vi "FPGA_ScanningPreview.vi"() -> ()   [LabVIEW 2024]
uses:
  <vilib>/rvi/Emulation/niFpgaSctlEmulationGetInTimedLoop.vi
  <vilib>/rvi/Emulation/niFpgaProcessEmulError.vi
  <vilib>/rvi/eio/common/nirviEmuTemplateMethod_errors.vi
  <vilib>/rvi/Emulation/niFpgaEmulationIsFPGAContextNoSignature.vi
  <vilib>/rvi/DataTransferAndStorage/Container/Common/niFpgaContainerGetUniqueNameForEmu.vi
  <vilib>/rvi/Memory/Memory_Emulation/niFpgaMemoryEmulationCacheClearOnFirstRun.vi
  <vilib>/rvi/Memory/Memory_Emulation/nirvimemoryEmulationManagerCache_MakeExclusive.vi
  <vilib>/rvi/Memory/Memory_Emulation/niFpgaMemoryEmulationValidateCache.vi
  <vilib>/rvi/Memory/Memory_Emulation/nirvimemoryEmulationManagerCache_InsertValue.vi
  <vilib>/Utility/error.llb/Clear Errors.vi
  <vilib>/rvi/Memory/Memory_Emulation/nirvimemoryEmulationManagerCache_ReleaseExclusive.vi
  <vilib>/rvi/Memory/Memory_Emulation/nirvimemoryEmulationManagerCache_GetValue.vi
  <vilib>/rvi/Memory/Memory_Emulation/nirvimemoryEmulationManagerCache_SetValue.vi
  <vilib>/rvi/Emulation/niFpgaGetClockAttributes.vi
  <vilib>/rvi/Emulation/niFpgaEmulationReportErrorSimple.vi
  <vilib>/rvi/Emulation/niFpgaCriticalErrorInLSC.vi
  <vilib>/eio/EIONode/EIONode.xnode
  <vilib>/rvi/DataTransferAndStorage/Container/XNode/niFpgaContainer.xnode
  <vilib>/rvi/DataTransferAndStorage/Register/Emulation/niFpgaRegisterEmulation.vi
  <vilib>/rvi/FXPMathLib/FxpAdd/XNode/nifxpmath_Add.xnode
  <vilib>/rvi/FXPMathLib/FxpSub/XNode/nifxpmath_Sub.xnode
  <vilib>/rvi/FXPMathLib/sim/FxpSim.dll
panel:
  in  "rate us":i32
  out "TargetDone?":bool
  out "ScanFinished?":bool
  in  "stop":bool
  in  "Y_end":fxp<+/-,48,16>
  in  "Y_start":fxp<+/-,48,16>
  in  "X_end":fxp<+/-,48,16>
  in  "X_start":fxp<+/-,48,16>
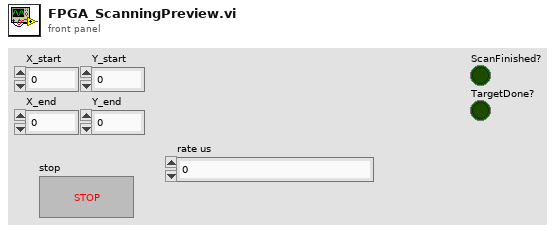
[diagram p1: front panel]
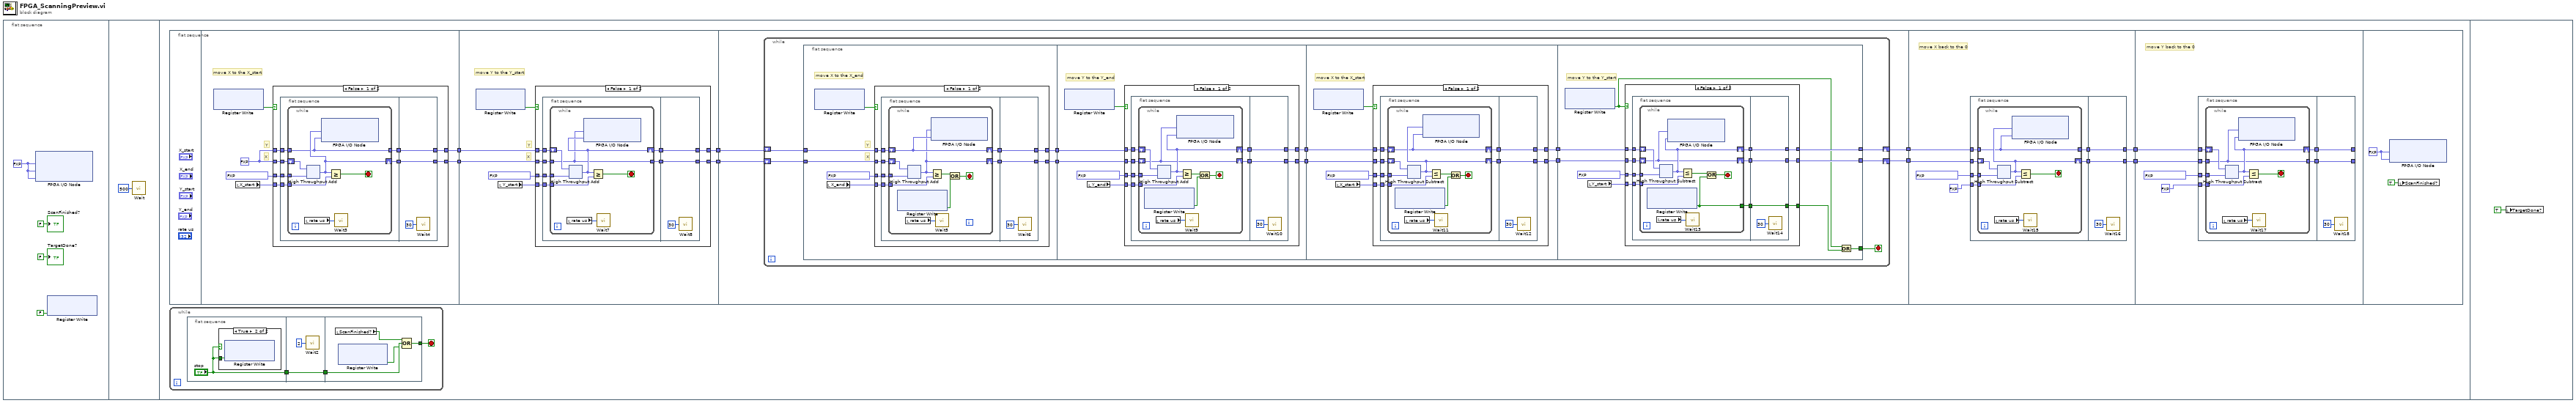
[diagram p0: block diagram]
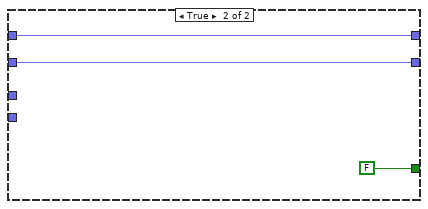
[diagram p8: hidden frame]
diagram:
  n1 = flat-sequence {
    frame #0 {
      w4 = fxp<+/-,20,5> 0.0 ("Connector0/AO0")
      n2 = xnode "FPGA I/O Node"("Connector0/AO0"=w4, "Connector0/AO1"=w4, "Connector0/AO2"=w4) -> ()  [unwired: 3 in, 3 out]
      n3 = xnode ("Register Write")("Data"=FALSE) -> ()  [unwired: 1 in, 1 out]
      "ScanFinished?" <- FALSE
      "TargetDone?" <- FALSE
    }
    frame #1 {
      n4 = call "Wait"("Count(mSec)"=u16 500) -> ()  [unwired: 1 out]
    }
    frame #2 {
      n5 = flat-sequence {
        tunnel: [w27] -> w13
        tunnel: [w25] -> w11
        tunnel: w13 -> [w59]
        tunnel: [w57] -> w12
        tunnel: w11 -> [w60]
        tunnel: [w58] -> w10
        tunnel: w10 -> [w93]
        tunnel: w12 -> [w92]
        tunnel: [w91] -> w9
        tunnel: [w90] -> w8
        tunnel: w9 -> [w258]
        tunnel: w8 -> [w257]
        tunnel: [w254] -> w7
        tunnel: [w253] -> w6
        tunnel: w7 -> [w278]
        tunnel: w6 -> [w277]
        frame #0 {
        }
        frame #1 {
          w26 = fxp<+/-,48,16> 0.0 ("y")
          # "X"
          # "Y"
          # "move X to the X_start"
          n6 = xnode ("Register Write")() -> ("Data"=w30:bool)  [unwired: 1 in, 1 out]
          n7 = local read "X_start"() -> (w28:fxp<+/-,48,16>)
          n8 = case shown="False" w30 {
            tunnel: w26 -> [w38 w56]
            tunnel: fxp<+/-,48,16> 0.00030517578125 ("y") -> [w37 _]
            tunnel: w28 -> [w36 _]
            tunnel: [w34 w56] -> w27
            tunnel: w26 -> [w33 w55]
            tunnel: [w31 w55] -> w25
            frame False {
              n9 = flat-sequence {
                tunnel: w38 -> [w42]
                tunnel: w37 -> [w44]
                tunnel: w36 -> [w43]
                tunnel: [w41] -> w35
                tunnel: w33 -> [w40]
                tunnel: [w39] -> w32
                tunnel: w35 -> [w53]
                tunnel: [w53] -> w34
                tunnel: w32 -> [w52]
                tunnel: [w52] -> w31
                frame #0 {
                  n10 = while {
                    tunnel: w44 -> [w51]
                    tunnel: w43 -> [w50]
                    shift-right: [w47] -> w41
                    shift-left: w42 -> [w48]
                    tunnel: w40 -> [w45]
                    tunnel: [w45] -> w39
                    stop <- w46 stop-if-true
                    n11 = local read "rate us"() -> (w49:i32)
                    n12 = xnode ("High Throughput Add")("x"=w48, "y"=w51) -> ("x+y"=w47:fxp<+/-,48,16>)
                    n13 = xnode "FPGA I/O Node"("Connector0/AO0"=w47, "Connector0/AO1"=w45) -> ()  [unwired: 2 in, 2 out]
                    n14 = Greater Or Equal?(x=w47, y=w50) -> (x >= y?=w46:bool)
                    n15 = call "Wait3"("Count(uSec)"=w49) -> ()  [unwired: 1 out]
                  }
                }
                frame #1 {
                  n16 = call "Wait4"("Count(uSec)"=u8 30) -> ()  [unwired: 1 out]
                }
              }
            }
            frame True {
            }
          }
        }
        frame #2 {
          # "X"
          # "Y"
          # "move Y to the Y_start"
          n17 = xnode ("Register Write")() -> ("Data"=w61:bool)  [unwired: 1 in, 1 out]
          n18 = local read "Y_start"() -> (w63:fxp<+/-,48,16>)
          n19 = case shown="False" w61 {
            tunnel: w59 -> [w71 w89]
            tunnel: fxp<+/-,48,16> 0.00030517578125 ("y") -> [w70 _]
            tunnel: w63 -> [w69 _]
            tunnel: [w67 w89] -> w57
            tunnel: w60 -> [w66 w88]
            tunnel: [w64 w88] -> w58
            frame False {
              n20 = flat-sequence {
                tunnel: w71 -> [w75]
                tunnel: w70 -> [w77]
                tunnel: w69 -> [w76]
                tunnel: [w74] -> w68
                tunnel: w66 -> [w73]
                tunnel: [w72] -> w65
                tunnel: w68 -> [w86]
                tunnel: [w86] -> w67
                tunnel: w65 -> [w85]
                tunnel: [w85] -> w64
                frame #0 {
                  n21 = while {
                    tunnel: w77 -> [w84]
                    tunnel: w76 -> [w83]
                    tunnel: w75 -> [w78]
                    tunnel: [w78] -> w74
                    shift-right: [w79] -> w72
                    shift-left: w73 -> [w81]
                    stop <- w80 stop-if-true
                    n22 = local read "rate us"() -> (w82:i32)
                    n23 = xnode ("High Throughput Add")("x"=w81, "y"=w84) -> ("x+y"=w79:fxp<+/-,48,16>)
                    n24 = xnode "FPGA I/O Node"("Connector0/AO0"=w78, "Connector0/AO1"=w79) -> ()  [unwired: 2 in, 2 out]
                    n25 = Greater Or Equal?(x=w79, y=w83) -> (x >= y?=w80:bool)
                    n26 = call "Wait7"("Count(uSec)"=w82) -> ()  [unwired: 1 out]
                  }
                }
                frame #1 {
                  n27 = call "Wait8"("Count(uSec)"=u8 30) -> ()  [unwired: 1 out]
                }
              }
            }
            frame True {
            }
          }
        }
        frame #3 {
          n28 = while {
            shift-right: [w95] -> w90
            shift-left: w92 -> [w101]
            shift-right: [w96] -> w91
            shift-left: w93 -> [w102]
            stop <- w94 stop-if-true
            n29 = flat-sequence {
              tunnel: w102 -> [w108]
              tunnel: w101 -> [w107]
              tunnel: [w106] -> w104
              tunnel: [w105] -> w103
              tunnel: w104 -> [w143]
              tunnel: w103 -> [w142]
              tunnel: [w141] -> w100
              tunnel: [w140] -> w99
              tunnel: w100 -> [w178]
              tunnel: w99 -> [w177]
              tunnel: [w176] -> w98
              tunnel: [w175] -> w97
              tunnel: w98 -> [w216]
              tunnel: w97 -> [w215]
              tunnel: [w214] -> w96
              tunnel: [w213] -> w95
              tunnel: [w210] -> w94
              frame #0 {
                # "X"
                # "Y"
                # "move X to the X_end"
                n30 = xnode ("Register Write")() -> ("Data"=w109:bool)  [unwired: 1 in, 1 out]
                n31 = local read "X_end"() -> (w111:fxp<+/-,48,16>)
                n32 = case shown="False" w109 {
                  tunnel: w107 -> [w119 w139]
                  tunnel: fxp<+/-,48,16> 0.00030517578125 ("y") -> [w118 _]
                  tunnel: w111 -> [w117 _]
                  tunnel: [w115 w139] -> w105
                  tunnel: w108 -> [w114 w138]
                  tunnel: [w112 w138] -> w106
                  frame False {
                    n33 = flat-sequence {
                      tunnel: w119 -> [w123]
                      tunnel: w118 -> [w125]
                      tunnel: w117 -> [w124]
                      tunnel: [w122] -> w116
                      tunnel: w114 -> [w121]
                      tunnel: [w120] -> w113
                      tunnel: w116 -> [w136]
                      tunnel: [w136] -> w115
                      tunnel: w113 -> [w135]
                      tunnel: [w135] -> w112
                      frame #0 {
                        n34 = while {
                          tunnel: w125 -> [w134]
                          tunnel: w124 -> [w133]
                          shift-right: [w126] -> w122
                          shift-left: w123 -> [w131]
                          shift-right: [w130] -> w120
                          shift-left: w121 -> [w130]
                          stop <- w127 stop-if-true
                          n35 = xnode ("Register Write")() -> ("Data"=w128:bool)  [unwired: 1 in, 1 out]
                          n36 = local read "rate us"() -> (w132:i32)
                          n37 = xnode ("High Throughput Add")("x"=w131, "y"=w134) -> ("x+y"=w126:fxp<+/-,48,16>)
                          n38 = Greater Or Equal?(x=w126, y=w133) -> (x >= y?=w129:bool)
                          n39 = xnode "FPGA I/O Node"("Connector0/AO0"=w126, "Connector0/AO1"=w130) -> ()  [unwired: 2 in, 2 out]
                          n40 = call "Wait5"("Count(uSec)"=w132) -> ()  [unwired: 1 out]
                          n41 = Or(x=w129, y=w128) -> (x .or. y?=w127:bool)
                        }
                      }
                      frame #1 {
                        n42 = call "Wait6"("Count(uSec)"=u8 30) -> ()  [unwired: 1 out]
                      }
                    }
                  }
                  frame True {
                  }
                }
              }
              frame #1 {
                # "move Y to the Y_end"
                n43 = xnode ("Register Write")() -> ("Data"=w146:bool)  [unwired: 1 in, 1 out]
                n44 = local read "Y_end"() -> (w144:fxp<+/-,48,16>)
                n45 = case shown="False" w146 {
                  tunnel: w142 -> [w154 w174]
                  tunnel: fxp<+/-,48,16> 0.00030517578125 ("y") -> [w153 _]
                  tunnel: w144 -> [w152 _]
                  tunnel: [w150 w174] -> w140
                  tunnel: w143 -> [w149 w173]
                  tunnel: [w147 w173] -> w141
                  frame False {
                    n46 = flat-sequence {
                      tunnel: w154 -> [w158]
                      tunnel: w153 -> [w160]
                      tunnel: w152 -> [w159]
                      tunnel: [w157] -> w151
                      tunnel: w149 -> [w156]
                      tunnel: [w155] -> w148
                      tunnel: w151 -> [w171]
                      tunnel: [w171] -> w150
                      tunnel: w148 -> [w170]
                      tunnel: [w170] -> w147
                      frame #0 {
                        n47 = while {
                          tunnel: w160 -> [w169]
                          tunnel: w159 -> [w168]
                          shift-right: [w165] -> w155
                          shift-left: w156 -> [w166]
                          shift-right: [w164] -> w157
                          shift-left: w158 -> [w164]
                          stop <- w161 stop-if-true
                          n48 = xnode ("Register Write")() -> ("Data"=w162:bool)  [unwired: 1 in, 1 out]
                          n49 = local read "rate us"() -> (w167:i32)
                          n50 = xnode ("High Throughput Add")("x"=w166, "y"=w169) -> ("x+y"=w165:fxp<+/-,48,16>)
                          n51 = xnode "FPGA I/O Node"("Connector0/AO0"=w164, "Connector0/AO1"=w165) -> ()  [unwired: 2 in, 2 out]
                          n52 = Greater Or Equal?(x=w165, y=w168) -> (x >= y?=w163:bool)
                          n53 = call "Wait9"("Count(uSec)"=w167) -> ()  [unwired: 1 out]
                          n54 = Or(x=w163, y=w162) -> (x .or. y?=w161:bool)
                        }
                      }
                      frame #1 {
                        n55 = call "Wait10"("Count(uSec)"=u8 30) -> ()  [unwired: 1 out]
                      }
                    }
                  }
                  frame True {
                  }
                }
              }
              frame #2 {
                # "move X to the X_start"
                n56 = xnode ("Register Write")() -> ("Data"=w179:bool)  [unwired: 1 in, 1 out]
                n57 = local read "X_start"() -> (w181:fxp<+/-,48,16>)
                n58 = case shown="False" w179 {
                  tunnel: w177 -> [w189 w209]
                  tunnel: fxp<+/-,48,16> 0.00030517578125 ("y") -> [w188 _]
                  tunnel: w181 -> [w187 _]
                  tunnel: [w185 w209] -> w175
                  tunnel: w178 -> [w184 w208]
                  tunnel: [w182 w208] -> w176
                  frame False {
                    n59 = flat-sequence {
                      tunnel: w189 -> [w193]
                      tunnel: w188 -> [w195]
                      tunnel: w187 -> [w194]
                      tunnel: [w192] -> w186
                      tunnel: w184 -> [w191]
                      tunnel: [w190] -> w183
                      tunnel: w186 -> [w206]
                      tunnel: [w206] -> w185
                      tunnel: w183 -> [w205]
                      tunnel: [w205] -> w182
                      frame #0 {
                        n60 = while {
                          tunnel: w195 -> [w201]
                          tunnel: w194 -> [w204]
                          shift-right: [w200] -> w192
                          shift-left: w193 -> [w202]
                          shift-right: [w199] -> w190
                          shift-left: w191 -> [w199]
                          stop <- w196 stop-if-true
                          n61 = xnode ("Register Write")() -> ("Data"=w197:bool)  [unwired: 1 in, 1 out]
                          n62 = local read "rate us"() -> (w203:i32)
                          n63 = xnode "High Throughput Subtract"("x"=w202, "y"=w201) -> ("x-y"=w200:fxp<+/-,48,16>)
                          n64 = xnode "FPGA I/O Node"("Connector0/AO0"=w200, "Connector0/AO1"=w199) -> ()  [unwired: 2 in, 2 out]
                          n65 = Less Or Equal?(x=w200, y=w204) -> (x <= y?=w198:bool)
                          n66 = call "Wait11"("Count(uSec)"=w203) -> ()  [unwired: 1 out]
                          n67 = Or(x=w198, y=w197) -> (x .or. y?=w196:bool)
                        }
                      }
                      frame #1 {
                        n68 = call "Wait12"("Count(uSec)"=u8 30) -> ()  [unwired: 1 out]
                      }
                    }
                  }
                  frame True {
                  }
                }
              }
              frame #3 {
                # "move Y to the Y_start"
                n69 = xnode ("Register Write")() -> ("Data"=w212:bool)  [unwired: 1 in, 1 out]
                n70 = local read "Y_start"() -> (w217:fxp<+/-,48,16>)
                n71 = case shown="False" w212 {
                  tunnel: w215 -> [w228 w251]
                  tunnel: fxp<+/-,48,16> 0.00030517578125 ("y") -> [w227 _]
                  tunnel: w217 -> [w226 _]
                  tunnel: [w224 w251] -> w213
                  tunnel: w216 -> [w223 w250]
                  tunnel: [w221 w250] -> w214
                  tunnel: [w219 FALSE ("Data")] -> w211
                  frame False {
                    n72 = flat-sequence {
                      tunnel: w228 -> [w233]
                      tunnel: w227 -> [w235]
                      tunnel: w226 -> [w234]
                      tunnel: [w232] -> w225
                      tunnel: w223 -> [w231]
                      tunnel: [w230] -> w222
                      tunnel: [w229] -> w220
                      tunnel: w225 -> [w247]
                      tunnel: [w247] -> w224
                      tunnel: w222 -> [w246]
                      tunnel: [w246] -> w221
                      tunnel: w220 -> [w245]
                      tunnel: [w245] -> w219
                      frame #0 {
                        n73 = while {
                          tunnel: w235 -> [w242]
                          tunnel: w234 -> [w244]
                          shift-right: [w240] -> w230
                          shift-left: w231 -> [w241]
                          tunnel: [w236] -> w229
                          shift-right: [w239] -> w232
                          shift-left: w233 -> [w239]
                          stop <- w237 stop-if-true
                          n74 = xnode ("Register Write")() -> ("Data"=w236:bool)  [unwired: 1 in, 1 out]
                          n75 = local read "rate us"() -> (w243:i32)
                          n76 = xnode "High Throughput Subtract"("x"=w241, "y"=w242) -> ("x-y"=w240:fxp<+/-,48,16>)
                          n77 = xnode "FPGA I/O Node"("Connector0/AO0"=w239, "Connector0/AO1"=w240) -> ()  [unwired: 2 in, 2 out]
                          n78 = Less Or Equal?(x=w240, y=w244) -> (x <= y?=w238:bool)
                          n79 = call "Wait13"("Count(uSec)"=w243) -> ()  [unwired: 1 out]
                          n80 = Or(x=w238, y=w236) -> (x .or. y?=w237:bool)
                        }
                      }
                      frame #1 {
                        n81 = call "Wait14"("Count(uSec)"=u8 30) -> ()  [unwired: 1 out]
                      }
                    }
                  }
                  frame True {
                  }
                }
                n82 = Or(x=w212, y=w211) -> (x .or. y?=w210:bool)
              }
            }
          }
        }
        frame #4 {
          # "move X back to the 0"
          n83 = flat-sequence {
            tunnel: w257 -> [w263]
            tunnel: fxp<+/-,48,16> 0.00030517578125 ("y") -> [w265]
            tunnel: fxp<+/-,48,16> 0.0 ("y") -> [w264]
            tunnel: [w262] -> w256
            tunnel: w258 -> [w261]
            tunnel: [w260] -> w255
            tunnel: w256 -> [w274]
            tunnel: [w274] -> w253
            tunnel: w255 -> [w273]
            tunnel: [w273] -> w254
            frame #0 {
              n84 = while {
                tunnel: w265 -> [w269]
                tunnel: w264 -> [w272]
                shift-right: [w267] -> w262
                shift-left: w263 -> [w270]
                tunnel: w261 -> [w266]
                tunnel: [w266] -> w260
                stop <- w268 stop-if-true
                n85 = local read "rate us"() -> (w271:i32)
                n86 = xnode "High Throughput Subtract"("x"=w270, "y"=w269) -> ("x-y"=w267:fxp<+/-,48,16>)
                n87 = xnode "FPGA I/O Node"("Connector0/AO0"=w267, "Connector0/AO1"=w266) -> ()  [unwired: 2 in, 2 out]
                n88 = Less Or Equal?(x=w267, y=w272) -> (x <= y?=w268:bool)
                n89 = call "Wait15"("Count(uSec)"=w271) -> ()  [unwired: 1 out]
              }
            }
            frame #1 {
              n90 = call "Wait16"("Count(uSec)"=u8 30) -> ()  [unwired: 1 out]
            }
          }
        }
        frame #5 {
          # "move Y back to the 0"
          n91 = flat-sequence {
            tunnel: w277 -> [w285]
            tunnel: fxp<+/-,48,16> 0.00030517578125 ("y") -> [w287]
            tunnel: fxp<+/-,48,16> 0.0 ("y") -> [w286]
            tunnel: [w284] -> w281
            tunnel: w278 -> [w283]
            tunnel: [w282] -> w280
            tunnel: w281 -> [w296]
            tunnel: [w296] -> _
            tunnel: w280 -> [w295]
            tunnel: [w295] -> _
            frame #0 {
              n92 = while {
                tunnel: w287 -> [w292]
                tunnel: w286 -> [w294]
                tunnel: w285 -> [w288]
                tunnel: [w288] -> w284
                shift-right: [w289] -> w282
                shift-left: w283 -> [w291]
                stop <- w290 stop-if-true
                n93 = local read "rate us"() -> (w293:i32)
                n94 = xnode "High Throughput Subtract"("x"=w291, "y"=w292) -> ("x-y"=w289:fxp<+/-,48,16>)
                n95 = xnode "FPGA I/O Node"("Connector0/AO0"=w288, "Connector0/AO1"=w289) -> ()  [unwired: 2 in, 2 out]
                n96 = Less Or Equal?(x=w289, y=w294) -> (x <= y?=w290:bool)
                n97 = call "Wait17"("Count(uSec)"=w293) -> ()  [unwired: 1 out]
              }
            }
            frame #1 {
              n98 = call "Wait18"("Count(uSec)"=u8 30) -> ()  [unwired: 1 out]
            }
          }
        }
        frame #6 {
          w299 = fxp<+/-,20,5> 0.0 ("Connector0/AO0")
          n99 = xnode "FPGA I/O Node"("Connector0/AO0"=w299, "Connector0/AO1"=w299) -> ()  [unwired: 2 in, 2 out]
          n100 = local write "ScanFinished?"(TRUE ("ScanFinished?")) -> ()
        }
      }
      n101 = while {
        stop <- w14 stop-if-true
        n102 = flat-sequence {
          tunnel: ["stop"] -> w16
          tunnel: w16 -> [w19]
          tunnel: [w19] -> w15
          tunnel: w15 -> [w23]
          tunnel: [w22] -> w14
          frame #0 {
            n103 = case shown="True" "stop" {
              tunnel: "stop" -> [_ w18]
              frame False {
              }
              frame True {
                n104 = xnode ("Register Write")("Data"=w18) -> ()  [unwired: 1 in, 1 out]
              }
            }
          }
          frame #1 {
            n105 = call "Wait2"("Count(mSec)"=u8 2 ("Count(uSec)")) -> ()  [unwired: 1 out]
          }
          frame #2 {
            n106 = local read "ScanFinished?"() -> (w24:bool)
            n107 = xnode ("Register Write")() -> ("Data"=w21:bool)  [unwired: 1 in, 1 out]
            n108 = Compound Arithmetic op=OR(w24, w23, w21) -> (w22:bool)
          }
        }
      }
    }
    frame #3 {
      n109 = local write "TargetDone?"(TRUE ("ScanFinished?")) -> ()
    }
  }
